vi "getbuffer.vi"(8 "error in":errorcluster, 9 "buffer size":u64, 10 "buffer name":string, 11 "Buffers":T1[](array[typedef])) -> (0 "error out":errorcluster, 1 "is locked":bool, 2 "output buffer":T1, 3 "Buffers out":T1[](array[typedef]), 5 "index":i32)   [LabVIEW 2016]
uses:
  private/vis/BufferStruct.ctl
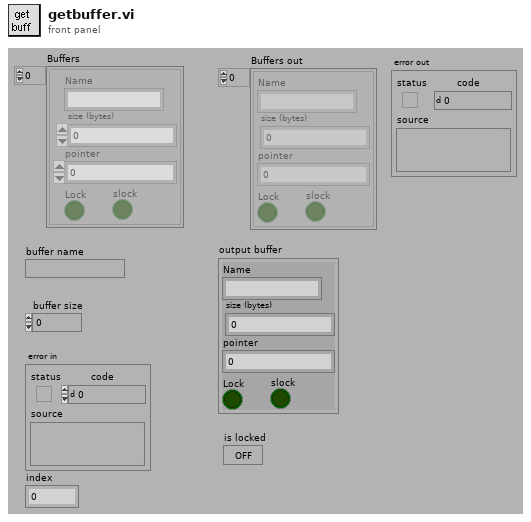
[diagram p1: front panel]
types:
  T1 = typedef "BufferStruct.ctl" = cluster{"Name":string, "size (bytes)":u64, "pointer":u64, "Lock":bool, "slock":bool}
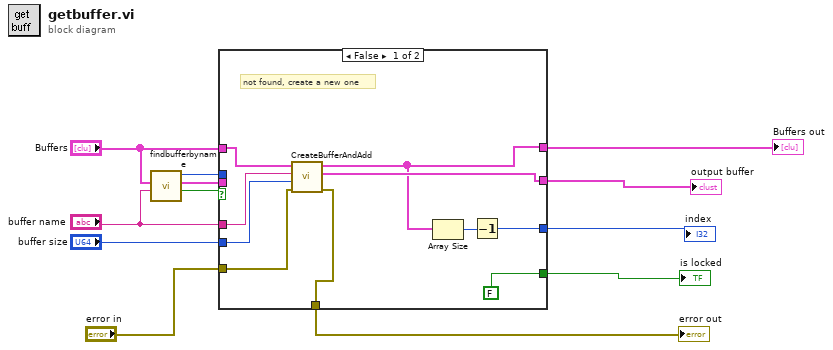
[diagram p0: block diagram]
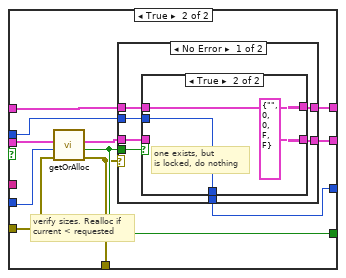
[diagram p2: hidden frame]
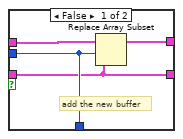
[diagram p3: hidden frame]
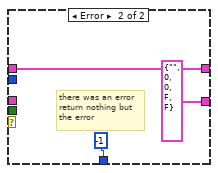
[diagram p4: hidden frame]
diagram:
  n1 = call "findbufferbyname.vi"("buffer name"="buffer name", "Buffers"="Buffers") -> ("found"=w3:bool, "buffer found"=w4:T1, "index"=w2:i32)  [unwired: 7 out]
  n2 = case shown="False" w3 {
    tunnel: w4 -> [_ w33]
    tunnel: "buffer size" -> [w19 w32]
    tunnel: "buffer name" -> [w20 _]
    tunnel: "Buffers" -> [w21 w31]
    tunnel: [w15 w28] -> w8
    tunnel: w2 -> [_ w29]
    tunnel: [w16 w23] -> w9
    tunnel: [FALSE ("is locked") w27] -> w10
    tunnel: "error in" -> [w18 w26]
    tunnel: [w17 w25] -> w12
    tunnel: [w13 w24] -> w1
    frame False {
      # "not found, create a new one"
      n3 = call "CreateBufferAndAdd.vi"("error in (no error)"=w18, "Size in Bytes"=w19, "Buffer Name"=w20, "Buffers"=w21) -> ("error out"=w17:errorcluster, "output buffer"=w16:T1, "output buffers"=w15:T1[])  [unwired: 5 out]
      n4 = Array Size(array=w15) -> (size(s)=w14:i32)
      n5 = Decrement(x=w14) -> (x-1=w13:i32)
    }
    frame True {
      # "verify sizes. Realloc if \ncurrent < requested"
      n6 = call "getOrAlloc.vi"("error in (no error)"=w26, "requested size"=w32, "current buffer"=w33) -> ("error out"=w25:errorcluster, "is locked"=w27:bool, "output buffer"=w30:T1)  [unwired: 6 out]
      n7 = case shown="No Error" w25 {
        tunnel: w31 -> [w40 w50]
        tunnel: w30 -> [w39 _]
        tunnel: w29 -> [w38 _]
        tunnel: [w37 w50] -> w28
        tunnel: w27 -> [w36 _]
        tunnel: [w35 T1 {"Name"="", "size (bytes)"=0, "pointer"=0, "Lock"=FALSE, "slock"=FALSE} ("output buffer")] -> w23
        tunnel: [w34 -1 ("index")] -> w24
        frame No Error {
          n8 = case shown="True" w36 {
            tunnel: w40 -> [w44 w47]
            tunnel: w39 -> [w41 _]
            tunnel: w38 -> [w42 w46]
            tunnel: [w43 w47] -> w37
            tunnel: [w41 T1 {"Name"="", "size (bytes)"=0, "pointer"=0, "Lock"=FALSE, "slock"=FALSE} ("output buffer")] -> w35
            tunnel: [w42 w46] -> w34
            frame False {
              # "add the new buffer"
              n9 = Replace Array Subset(array=w44, new element=w41, index=w42) -> (w43:T1[])
            }
            frame True {
              # "one exists, but\nis locked, do nothing"
            }
          }
        }
        frame Error {
          # "there was an error\nreturn nothing but\nthe error"
        }
      }
    }
  }
  "error out" <- w12
  "is locked" <- w10
  "output buffer" <- w9
  "Buffers out" <- w8
  "index" <- w1
